vi "Make Shot Directory.vi"(0 "daily test directory":path) -> (7 "shot directory":path, 10 "error out":errorcluster)   [LabVIEW 2018]
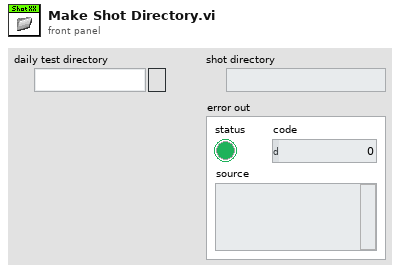
[diagram p1: front panel]
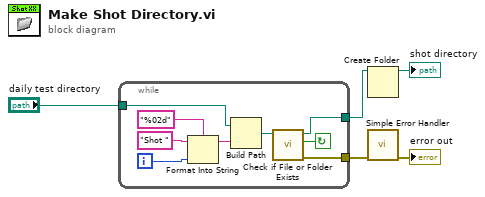
[diagram p0: block diagram]
diagram:
  n1 = while {
    tunnel: "daily test directory" -> [w12]
    tunnel: [w8] -> w1
    tunnel: [w6] -> w2
    i -> [w9]
    stop <- w7 continue-if-true
    n2 = Format Into String(format string="%02d", initial string="Shot ", w9) -> (resulting string=w11:string)  [unwired: 1 in, 1 out]
    n3 = Build Path(base path=w12, name or relative path=w11) -> (appended path=w10:path)
    n4 = call <vilib>:"Check if File or Folder Exists.vi"("path"=w10) -> ("error out"=w6:errorcluster, "file or folder exists?"=w7:bool, "dup path"=w8:path)  [unwired: 8 in]
  }
  n5 = Create Folder(path (use dialog)=w1) -> (created path=→"shot directory":path)  [unwired: 2 in, 2 out]
  n6 = call <vilib>:"Simple Error Handler.vi"("error in (no error)"=w2) -> ("error out"=→"error out":errorcluster)  [unwired: 4 in, 4 out]
